vi "WritePressureToReport.vi"(8 "error in (no error)":errorcluster, 9 "LowPressure":bool, 10 "Initial":bool, 11 "isMylarTest":bool) -> (0 "error out":errorcluster)   [LabVIEW 2018, in "S1.lvclass"]
uses:
  S1.lvclass
  Public Controls/ReportHeader.ctl
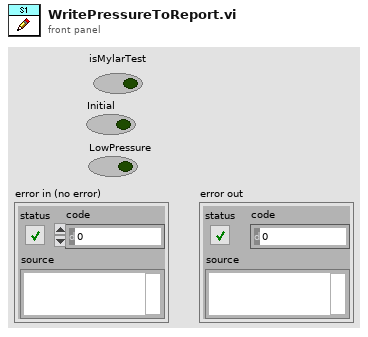
[diagram p1: front panel]
types:
  T1 = typedef "S1.lvclass/ReportHeader.ctl" = string
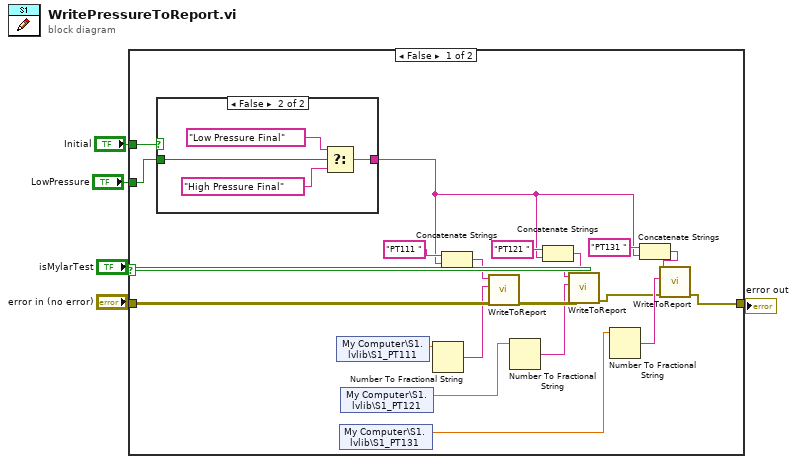
[diagram p0: block diagram]
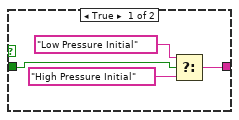
[diagram p2: hidden frame]
diagram:
  n1 = case shown="False" "isMylarTest" {
    tunnel: "error in (no error)" -> [w18 w33]
    tunnel: [w15 w33] -> w5
    tunnel: "LowPressure" -> [w11 _]
    tunnel: "Initial" -> [w12 _]
    frame False {
      n2 = case shown="False" w12 {
        tunnel: w11 -> [w26 w32]
        tunnel: [w25 w29] -> w6
        frame True {
          n3 = Select(t=T1 "Low Pressure Initial" ("Header"), s=w26, f=T1 "High Pressure Initial" ("Header")) -> (s? t:f=w25:T1)
        }
        frame False {
          n4 = Select(t=T1 "Low Pressure Final" ("Header"), s=w32, f=T1 "High Pressure Final" ("Header")) -> (s? t:f=w29:T1)
        }
      }
      n5 = shared-variable "My Computer\\S1.lvlib\\S1_PT111"() -> (w24:dbl)  [unwired: 1 in, 1 out]
      n6 = shared-variable "My Computer\\S1.lvlib\\S1_PT131"() -> (w19:dbl)  [unwired: 1 in, 1 out]
      n7 = shared-variable "My Computer\\S1.lvlib\\S1_PT121"() -> (w22:dbl)  [unwired: 1 in, 1 out]
      n8 = Number To Fractional String(number=w24) -> (F-format string=w23:string)  [unwired: 3 in]
      n9 = Concatenate Strings("PT111 " ("string"), w6) -> (w14:string)
      n10 = call "WriteToReport.vi"("error in"=w18, "Value"=w23, "Header"=w14) -> ("error out"=w17:errorcluster)  [unwired: 8 in]
      n11 = Number To Fractional String(number=w22) -> (F-format string=w21:string)  [unwired: 3 in]
      n12 = Concatenate Strings("PT121 " ("string"), w6) -> (w9:string)
      n13 = call "WriteToReport.vi"("error in"=w17, "Value"=w21, "Header"=w9) -> ("error out"=w16:errorcluster)  [unwired: 8 in]
      n14 = Number To Fractional String(number=w19) -> (F-format string=w20:string)  [unwired: 3 in]
      n15 = Concatenate Strings("PT131 " ("string"), w6) -> (w7:string)
      n16 = call "WriteToReport.vi"("error in"=w16, "Value"=w20, "Header"=w7) -> ("error out"=w15:errorcluster)  [unwired: 8 in]
    }
    frame True {
    }
  }
  "error out" <- w5
